vi "Tab Visibilities - Default--Const.vi"() -> (3 "Tab Visbility":bool[](array[boolean])=[TRUE, FALSE, FALSE, FALSE, FALSE, FALSE, FALSE])   [LabVIEW 2017, in "DTacq Plot Display Library.lvlib"]
uses:
  DTacq Plot Display Library.lvlib
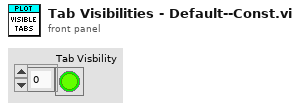
[diagram p1: front panel]
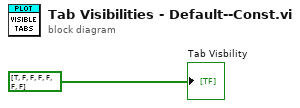
[diagram p0: block diagram]
diagram:
  "Tab Visbility" <- bool[] [TRUE, FALSE, FALSE, FALSE, FALSE, FALSE, FALSE]
